vi "Package Manager Path.vi"() -> (4 "Package Manager Path":path)   [LabVIEW 2021, in "Path Functions.lvlib"]
uses:
  Path Functions.lvlib
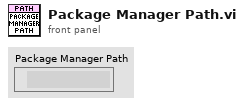
[diagram p1: front panel]
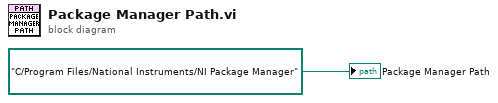
[diagram p0: block diagram]
diagram:
  "Package Manager Path" <- path "C:/Program Files/National Instruments/NI Package Manager" ("working directory")
